vi "Pasco Excel Write.vi"(5 "Folder Location":string, 7 "File Name":string, 8 "WriteToExcel":bool, 11 "2D data":dbl[][](array[numeric]) format="%0.2f") -> (3 "Sent?":string="File Wrote")   [LabVIEW 2011]
uses:
  <vilib>/Utility/file.llb/Write To Spreadsheet File (DBL).vi
panel:
  out "new file path (Not A Path if cancelled)":path
  out "path":path
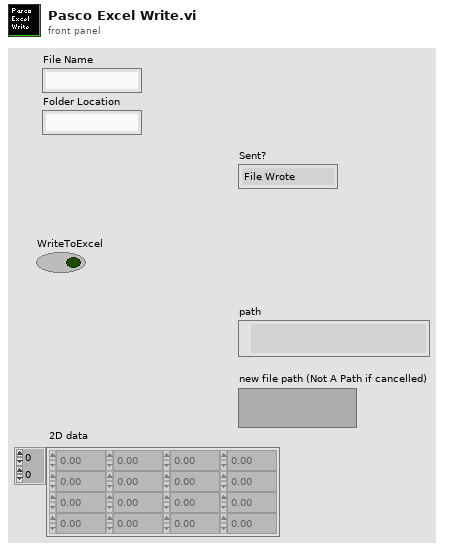
[diagram p1: front panel]
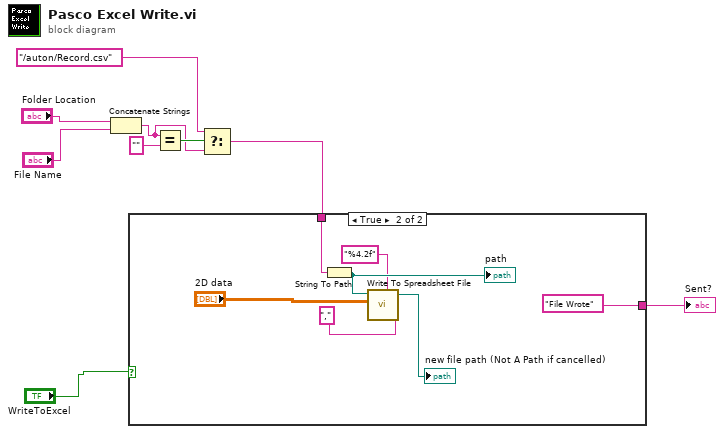
[diagram p0: block diagram]
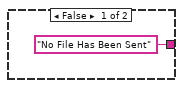
[diagram p2: hidden frame]
diagram:
  n1 = Concatenate Strings("Folder Location", "File Name") -> (w2:string)
  n2 = Equal?(x=w2, y="") -> (x = y?=w4:bool)
  n3 = Select(t="/auton/Record.csv" ("string"), s=w4, f=w2) -> (s? t:f=w1:string)
  n4 = case shown="True" "WriteToExcel" {
    tunnel: ["No File Has Been Sent" "File Wrote"] -> w8
    tunnel: w1 -> [_ w12]
    frame False {
    }
    frame True {
      n5 = String To Path(string=w12) -> (path=w17:path)
      "path" <- w17
      n6 = call-poly <vilib>:"Write To Spreadsheet File.vi"("delimiter (\\t)"="," ("delimiter (\\t)"), "format (%.3f)"="%4.2f", "2D data"="2D data", "file path (dialog if empty)"=w17) -> ("new file path (Not A Path if cancelled)"=→"new file path (Not A Path if cancelled)":path)  [unwired: 4 in]
    }
  }
  "Sent?" <- w8
